vi "Test.vi"() -> ()   [LabVIEW 2009]
uses:
  Tree/Tree.lvclass
  Tree/SearchMethod.ctl
  Waypoint/point.ctl
  Waypoint/Waypoint.lvclass
  RouteTree.lvclass
panel:
  out "Best First Distance":dbl
  out "greedy path":dbl
  out "greedy Path":T1[](array[typedef])
  out "2D Picture":picture
  in  "Number of Points":i32=5
  out "time":u32
  out "Best First Path":T1[](array[typedef])
  out "found":bool
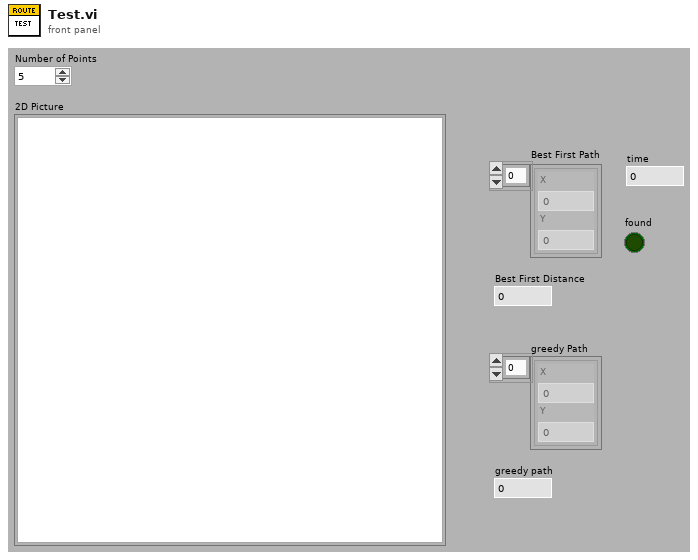
[diagram p1: front panel]
types:
  T1 = typedef "Waypoint.lvclass/point.ctl" = cluster{"X":dbl, "Y":dbl}
  T2 = typedef "Tree.lvclass/SearchMethod.ctl" = enum16{"Breadth (First)", "Depth (First)", "Best First", "Breadth (Exhaustive)", "Depth (Exhaustive)"}
  T3 = cluster{"Width":u16, "Style":enum32{"Solid", "Dash", "Dot", "DashDot", "DashDotDot"}}
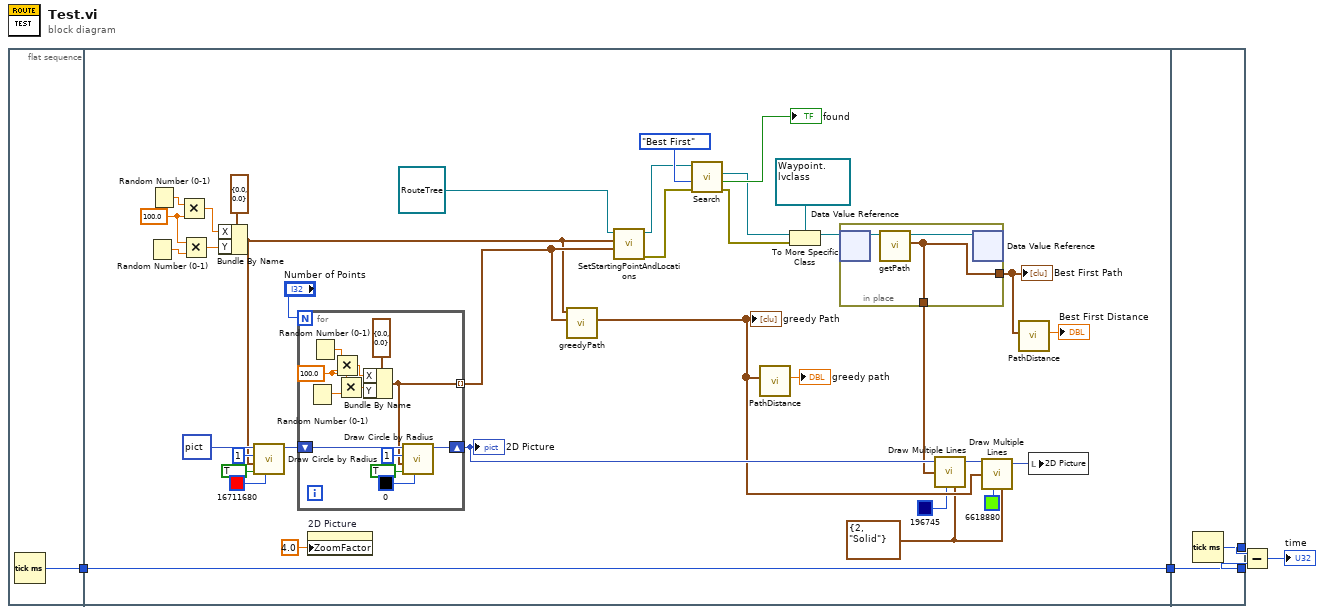
[diagram p0: block diagram]
diagram:
  n1 = flat-sequence {
    tunnel: [w6] -> w5
    tunnel: w5 -> [w34]
    tunnel: [w34] -> w4
    tunnel: [w59] -> w2
    tunnel: [w58] -> w3
    tunnel: w4 -> [w58]
    frame #0 {
      n2 = Tick Count (ms)() -> (millisecond timer value=w6:u32)
    }
    frame #1 {
      w7 = T3 {"Width"=2, "Style"=enum."Solid"} ("pen")
      w28 = 100.0 ("y")
      n3 = Random Number (0-1)() -> (number: 0 to 1=w29:dbl)
      n4 = Random Number (0-1)() -> (number: 0 to 1=w31:dbl)
      n5 = Multiply(x=w31, y=w28) -> (x*y=w30:dbl)
      n6 = Multiply(x=w28, y=w29) -> (x*y=w27:dbl)
      n7 = Bundle By Name(cluster=T1 {"X"=0.0, "Y"=0.0} ("point"), "X"=w30, "Y"=w27) -> (w17:T1)
      n8 = call <vilib>:"Draw Circle by Radius.vi"("color(black)"=u32 16711680, "fill?(F)"=TRUE, "pixel center"=w17, "radius"=i16 1, "picture"=picture data[5B] ("2D Picture")) -> ("new picture"=w21:picture)  [unwired: 6 in]
      n9 = for {
        N: "Number of Points" -> [_]
        tunnel: [w45] -> w18 mode=indexing
        shift-right: [w48] -> w25
        shift-left: w21 -> [w49]
        w50 = 100.0 ("x")
        n10 = Random Number (0-1)() -> (number: 0 to 1=w52:dbl)
        n11 = Random Number (0-1)() -> (number: 0 to 1=w54:dbl)
        n12 = Multiply(x=w54, y=w50) -> (x*y=w53:dbl)
        n13 = Multiply(x=w50, y=w52) -> (x*y=w51:dbl)
        n14 = Bundle By Name(cluster=T1 {"X"=0.0, "Y"=0.0} ("point"), "X"=w53, "Y"=w51) -> (w45:T1)
        n15 = call <vilib>:"Draw Circle by Radius.vi"("color(black)"=u32 0, "fill?(F)"=TRUE, "pixel center"=w45, "radius"=i16 1, "picture"=w49) -> ("new picture"=w48:picture)  [unwired: 6 in]
      }
      "2D Picture" <- w25
      n16 = property on="2D Picture" class="Pict"("ZoomFactor"=sgl 4.0 ("Zoom Factor")) -> ()  [unwired: 2 in, 2 out]
      n17 = call "greedyPath.vi"("ToVisit"=w18, "start"=w17) -> ("greedy Path"=w13:T1[])  [unwired: 8 in, 1 out]
      "greedy Path" <- w13
      n18 = call "SetStartingPointAndLocations.vi"("locations"=w18, "point"=w17, "PathTree in"=refnum<class "RouteTree.lvclass"> refnum ("PathTree.lvclass")) -> ("error out"=w40:errorcluster, "PathTree out"=w41:refnum<class "RouteTree.lvclass">)  [unwired: 7 in]
      n19 = call "Search.vi"("error in (no error)"=w40, "SearchMethod"=SearchMethod."Best First", "Tree in"=w41) -> ("error out"=w26:errorcluster, "found"=→"found":bool, "Node"=w36:refnum<data-value>)  [unwired: 5 in, 1 out]
      n20 = call "PathDistance.vi"("path"=w13) -> ("distance"=→"greedy path":dbl)  [unwired: 10 in]
      n21 = To More Specific Class(target class=refnum<data-value> refnum ("data value reference"), reference=w36, error in=w26) -> (specific class reference=w37:refnum<data-value>)  [unwired: 1 out]
      n22 = in-place {
        in-place-border: [w55] -> w11
        in-place-border: [w55] -> w24
        n23 = in-place-dvr #1(w37) -> (w57:refnum<class "Waypoint.lvclass">)  [unwired: 1 out]
        n24 = call "getPath.vi"("Waypoint in"=w57) -> ("Path"=w55:T1[], "Waypoint out"=w56:refnum<class "Waypoint.lvclass">)  [unwired: 8 in, 1 out]
        n25 = in-place-dvr #1(w56) -> ()  [unwired: 2 out]
      }
      "Best First Path" <- w11
      n26 = call <vilib>:"Draw Multiple Lines.vi"("picture"=w25, "line endpoints"=w24, "color(black)"=u32 196745, "pen"=w7) -> ("new picture"=w16:picture)  [unwired: 5 in]
      n27 = call <vilib>:"Draw Multiple Lines.vi"("picture"=w16, "line endpoints"=w13, "color(black)"=u32 6618880, "pen"=w7) -> ("new picture"=w15:picture)  [unwired: 5 in]
      n28 = call "PathDistance.vi"("path"=w11) -> ("distance"=→"Best First Distance":dbl)  [unwired: 10 in]
      n29 = local write "2D Picture"(w15) -> ()
    }
    frame #2 {
      n30 = Tick Count (ms)() -> (millisecond timer value=w59:u32)
    }
  }
  n31 = Subtract(x=w2, y=w3) -> (x-y=→"time":u32)
